vi "Create.vi"(8 "error in (no error)":errorcluster, 11 "count":i32) -> (0 "error out":errorcluster)   [LabVIEW 2017, in "McsaResourceScheduler.lvlib"]
uses:
  <vilib>/addons/InsightCM/Devices/Shared/Mcsa/McsaResourceScheduler/McsaResourceScheduler.lvlib
  <vilib>/addons/InsightCM/Devices/Shared/Mcsa/McsaResourceScheduler/controls/InternalAction.ctl
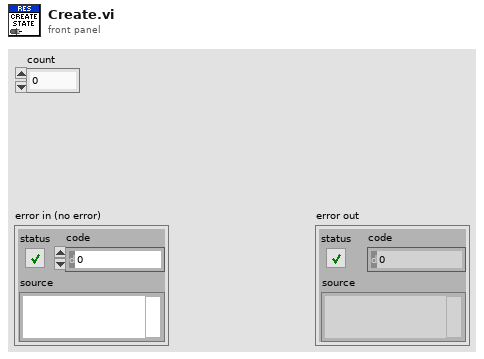
[diagram p1: front panel]
types:
  T1 = typedef "McsaResourceScheduler.lvlib/InternalAction.ctl" = enum16{"Initialize", "Register", "Unregister", "Get"}
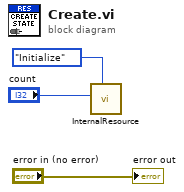
[diagram p0: block diagram]
diagram:
  n1 = call <vilib>:"InternalResource.vi"("action"=InternalAction."Initialize", "count"="count") -> ()  [unwired: 8 in, 2 out]
  "error out" <- "error in (no error)"
